vi "output.vi"(1 "input":T2) -> (0 "output":T1)   [LabVIEW 2013]
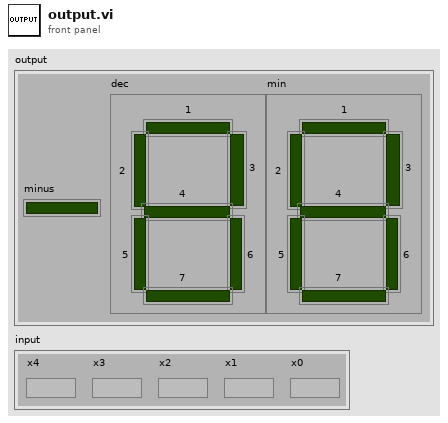
[diagram p1: front panel]
types:
  T1 = cluster{"minus":bool, "dec":cluster{"1":bool, "2":bool, "3":bool, "4":bool, "5":bool, "6":bool, "7":bool}, "min":cluster{"1":bool, "2":bool, "3":bool, "4":bool, "5":bool, "6":bool, "7":bool}}
  T2 = cluster{"x4":bool, "x3":bool, "x2":bool, "x1":bool, "x0":bool}
  T3 = cluster{"dec":cluster{"y3":bool, "y2":bool, "y1":bool, "y0":bool}, "min":cluster{"y3":bool, "y2":bool, "y1":bool, "y0":bool}}
  T4 = cluster{"y3":bool, "y2":bool, "y1":bool, "y0":bool}
  T5 = cluster{bool, "y3":bool, "y2":bool, "y1":bool, "y0":bool}
  T6 = cluster{"1":bool, "2":bool, "3":bool, "4":bool, "5":bool, "6":bool, "7":bool}
  T7 = cluster{"minus":bool, "output":cluster{"1":bool, "2":bool, "3":bool, "4":bool, "5":bool, "6":bool, "7":bool}, "output":cluster{"1":bool, "2":bool, "3":bool, "4":bool, "5":bool, "6":bool, "7":bool}}
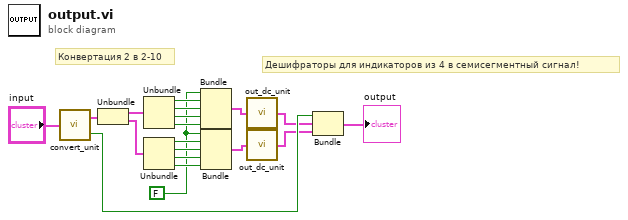
[diagram p0: block diagram]
diagram:
  w5 = FALSE
  # "Дешифраторы для индикаторов из 4 в семисегментный сигнал!"
  # "Конвертация 2 в 2-10"
  n1 = call "convert_unit.vi"("input"="input") -> ("output"=w16:T3, "minus"=w17:bool)
  n2 = Unbundle(w16) -> ("dec"=w15:T4, "min"=w14:T4)
  n3 = Unbundle(w15) -> ("y3"=w6:bool, "y2"=w7:bool, "y1"=w8:bool, "y0"=w9:bool)
  n4 = Unbundle(w14) -> ("y3"=w10:bool, "y2"=w11:bool, "y1"=w12:bool, "y0"=w13:bool)
  n5 = Bundle(w5, "y3"=w6, "y2"=w7, "y1"=w8, "y0"=w9) -> (w4:T5)  [unwired: 1 in]
  n6 = Bundle(w5, "y3"=w10, "y2"=w11, "y1"=w12, "y0"=w13) -> (w3:T5)  [unwired: 1 in]
  n7 = call "out_dc_unit.vi"("input"=w4) -> ("output"=w1:T6)
  n8 = call "out_dc_unit.vi"("input"=w3) -> ("output"=w2:T6)
  n9 = Bundle("minus"=w17, "output"=w1, "output"=w2) -> (→"output":T7)  [unwired: 1 in]
